vi "CommonVIs_GetClassObjectRefPath.vi"(1 "llbClassPath":path, 5 "error in (no error)":errorcluster) -> (15 "classObjectRefPath":path, 19 "error out":errorcluster)   [LabVIEW 2020]
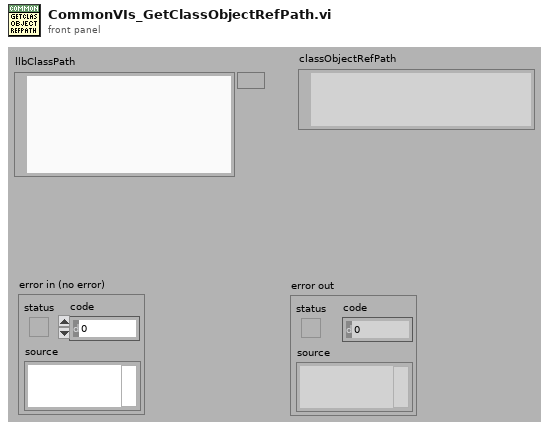
[diagram p1: front panel]
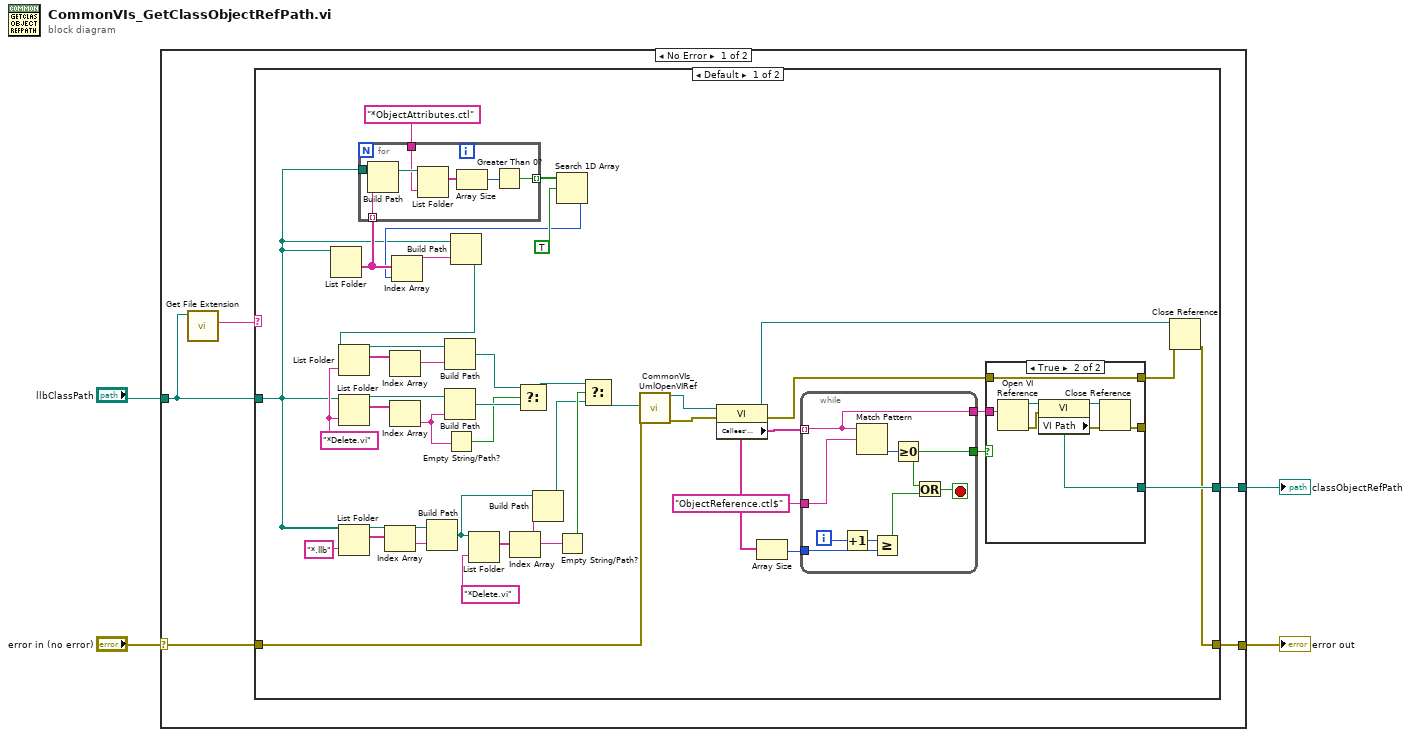
[diagram p0: block diagram]
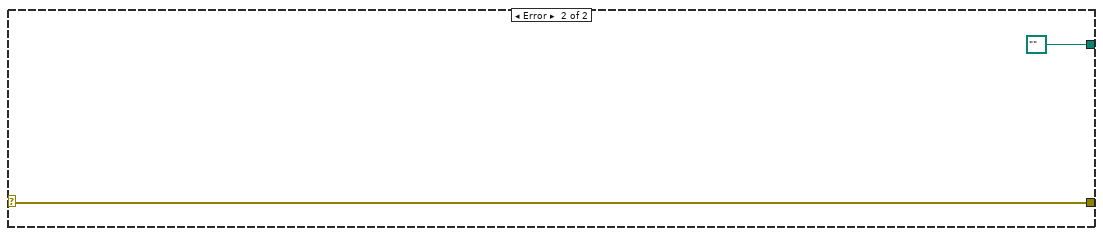
[diagram p4: hidden frame]
diagram:
  n1 = case shown="No Error" "error in (no error)" {
    selector: "error in (no error)" -> [w8 w80]
    tunnel: "llbClassPath" -> [w6 _]
    tunnel: [w7 path "" ("Path")] -> w1
    tunnel: [w9 w80] -> w3
    frame No Error {
      n2 = call <vilib>:"Get File Extension.vi"("file"=w6) -> ("lowercase file extension"=w5:string)  [unwired: 1 in, 9 out]
      n3 = case shown="Default" w5 {
        tunnel: [w14 w77] -> w9
        tunnel: w8 -> [w12 w77]
        tunnel: [w32 w78] -> w7
        tunnel: w6 -> [w15 w78]
        frame Default {
          w46 = "*Delete.vi" ("pattern")
          n4 = List Folder(path=w15) -> (folder names=w37:string[])  [unwired: 1 in, 5 out]
          n5 = List Folder(path=w15, pattern=w46) -> (path out=w51:path, filenames=w50:string[])  [unwired: 1 in, 3 out]
          n6 = List Folder(path=w15, pattern="*.llb") -> (filenames=w30:string[])  [unwired: 1 in, 4 out]
          n7 = for {
            tunnel: w37 -> [w75] mode=indexing
            tunnel: w15 -> [w76]
            tunnel: "*ObjectAttributes.ctl" ("string") -> [w73]
            tunnel: [w70] -> w39 mode=indexing
            n8 = Build Path(base path=w76, name or relative path=w75) -> (appended path=w74:path)
            n9 = List Folder(path=w74, pattern=w73) -> (filenames=w72:string[])  [unwired: 1 in, 4 out]
            n10 = Array Size(array=w72) -> (size(s)=w71:i32)
            n11 = Greater Than 0?(x=w71) -> (x > 0?=w70:bool)
          }
          n12 = Index Array(array=w30) -> (element=w29:string)  [unwired: 1 in]
          n13 = Index Array(array=w50) -> (element=w42:string)  [unwired: 1 in]
          n14 = Build Path(base path=w15, name or relative path=w29) -> (appended path=w26:path)
          n15 = Build Path(base path=w51, name or relative path=w42) -> (appended path=w44:path)
          n16 = Empty String/Path?(string/path=w42) -> (empty?=w41:bool)
          n17 = List Folder(path=w26, pattern="*Delete.vi" ("string")) -> (filenames=w27:string[])  [unwired: 1 in, 4 out]
          n18 = Index Array(array=w27) -> (element=w25:string)  [unwired: 1 in]
          n19 = Build Path(base path=w26, name or relative path=w25) -> (appended path=w22:path)
          n20 = Search 1D Array(1D array=w39, element=TRUE) -> (index of element=w36:i32)  [unwired: 1 out]
          n21 = Index Array(array=w37, index=w36) -> (element=w35:string)
          n22 = Build Path(base path=w15, name or relative path=w35) -> (appended path=w34:path)
          n23 = List Folder(path=w34, pattern=w46) -> (path out=w47:path, filenames=w48:string[])  [unwired: 1 in, 3 out]
          n24 = Index Array(array=w48) -> (element=w45:string)  [unwired: 1 in]
          n25 = Build Path(base path=w47, name or relative path=w45) -> (appended path=w43:path)
          n26 = Select(t=w43, s=w41, f=w44) -> (s? t:f=w23:path)
          n27 = Empty String/Path?(string/path=w25) -> (empty?=w24:bool)
          n28 = Select(t=w23, s=w24, f=w22) -> (s? t:f=w13:path)
          n29 = call "CommonVIs_UmlOpenVIRef.vi"("error in"=w12, "ViPath/ViName"=w13) -> ("error out"=w11:errorcluster, "vi reference"=w10:refnum<vi>)  [unwired: 2 in, 6 out]
          n30 = property class="VI"(reference=w10, error in=w11) -> (reference out=w49:refnum<vi>, error out=w16:errorcluster, "Callees' Names"=w21:string[])
          n31 = Array Size(array=w21) -> (size(s)=w20:i32)
          n32 = while {
            tunnel: w21 -> [w61] mode=indexing
            tunnel: w20 -> [w67]
            tunnel: "ObjectReference.ctl$" -> [w66]
            tunnel: [w64] -> w18
            tunnel: [w61] -> w17
            i -> [w69]
            stop <- w62 stop-if-true
            n33 = Increment(x=w69) -> (x+1=w68:i32)
            n34 = Match Pattern(string=w61, regular expression=w66) -> (offset past match=w65:i32)  [unwired: 4 out]
            n35 = Greater Or Equal?(x=w68, y=w67) -> (x >= y?=w63:bool)
            n36 = Greater Or Equal To 0?(x=w65) -> (x >= 0?=w64:bool)
            n37 = Or(x=w64, y=w63) -> (x .or. y?=w62:bool)
          }
          n38 = case shown="True" w18 {
            tunnel: w17 -> [_ w60]
            tunnel: w16 -> [w52 w55]
            tunnel: [w52 w55] -> w33
            tunnel: [_ w54] -> w32
            tunnel: [_ w53] -> _
            frame False {
            }
            frame True {
              n39 = Open VI Reference(vi path=w60) -> (vi reference=w59:refnum<vi>, error out=w58:errorcluster)  [unwired: 1 in, 4 out]
              n40 = property class="VI"(reference=w59, error in=w58) -> (reference out=w56:refnum<vi>, error out=w57:errorcluster, "VI Path"=w54:path)
              n41 = Close Reference(reference=w56, error in (no error)=w57) -> (error out=w53:errorcluster)
            }
          }
          n42 = Close Reference(reference=w49, error in (no error)=w33) -> (error out=w14:errorcluster)
        }
        frame "lvclass" {
        }
      }
    }
    frame Error {
    }
  }
  "error out" <- w3
  "classObjectRefPath" <- w1
